vi "GetProcessChanConfig.vi"(8 "error in":errorcluster, 10 "Channel Number":T1=1 items=["Channel 1"=1, "Channel 2"=2, "Channel 3"=3, "Channel 4"=4, "Channel 5"=5, "Channel 6"=6, "Channel 7"=7, "Channel 8"=8], 11 "VISA resource name":refnum<visa-resource-name>) -> (0 "error out":errorcluster, 2 "channel configuration information":string, 3 "VISA resource name out":refnum<visa-resource-name>)   [LabVIEW 2023, in "Thermotron 8800.lvlib"]
doc: "CCNF\nCommand name: Send process channel configuration information\nCommand type: System status\nDescription: The 8800 sends a single coded integer describing the channel type.\n0 = Channel not used\n1 = Percent relative humidity channel using a wet bulb/dry bulb thermocouple pair\n2 = Temperature channel using a thermocouple\n3 = Linear channel using a programmable range (for example altitude)\n4 = Linear 0% to 100% relative humidity channel using a solid-state sensor\n5 = Product temperature control channel\nSyntax: CCNFn?\nWhere n is any process variable channel (1 to 8).\nData type: Coded integer\nQuery example: CCNF2?\n8800 response: 4 (Linear % relative humidity)"
uses:
  Thermotron 8800.lvlib
  Private/AnalogInputChannelNumber.ctl
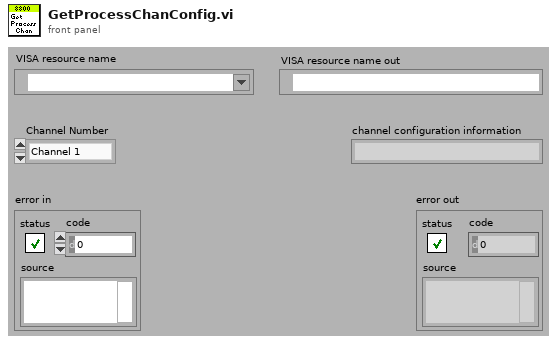
[diagram p1: front panel]
types:
  T1 = typedef "Thermotron 8800.lvlib/AnalogInputChannelNumber.ctl" = u16
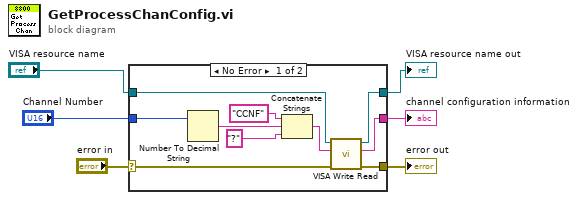
[diagram p0: block diagram]
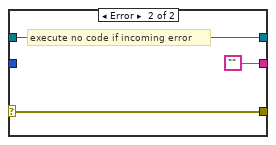
[diagram p2: hidden frame]
diagram:
  n1 = case shown="No Error" "error in" {
    selector: "error in" -> [w8 w18]
    tunnel: "Channel Number" -> [w13 _]
    tunnel: "VISA resource name" -> [w12 w19]
    tunnel: [w11 w19] -> w4
    tunnel: [w10 ""] -> w3
    tunnel: [w9 w18] -> w2
    frame No Error {
      n2 = Number To Decimal String(number=w13) -> (decimal integer string=w14:string)  [unwired: 1 in]
      n3 = Concatenate Strings("CCNF" ("8800 Command"), w14, "?" ("8800 Command")) -> (w15:string)
      n4 = call "VISA Write Read.vi"("error in (no error)"=w8, "8800 Command"=w15, "VISA Refnum in"=w12) -> ("error out"=w9:errorcluster, "read buffer"=w10:string, "VISA Refnum out"=w11:refnum<visa-resource-name>)  [unwired: 6 in]
    }
    frame Error {
      # "execute no code if incoming error"
    }
  }
  "VISA resource name out" <- w4
  "channel configuration information" <- w3
  "error out" <- w2
